vi "read_idcode.vi"() -> ()   [LabVIEW 2017]
panel:
  out "字符串":string
  out "数值":i32=2
  out "Out":u8=67 format="%.0x"
  out "received string 2":string="C"
  out "received string":string
  in  "数组":string[](array[string])=[":\u0005\u0000\u0000\u0000\u001f\u0000", ":\u0004\u0000\u0000\u0000\u0002\u0000", ": \u0000\u0000\u0000\u0000\u0000"]
  out "错误输出":errorcluster
  in  "address":string="192.168.10.20"
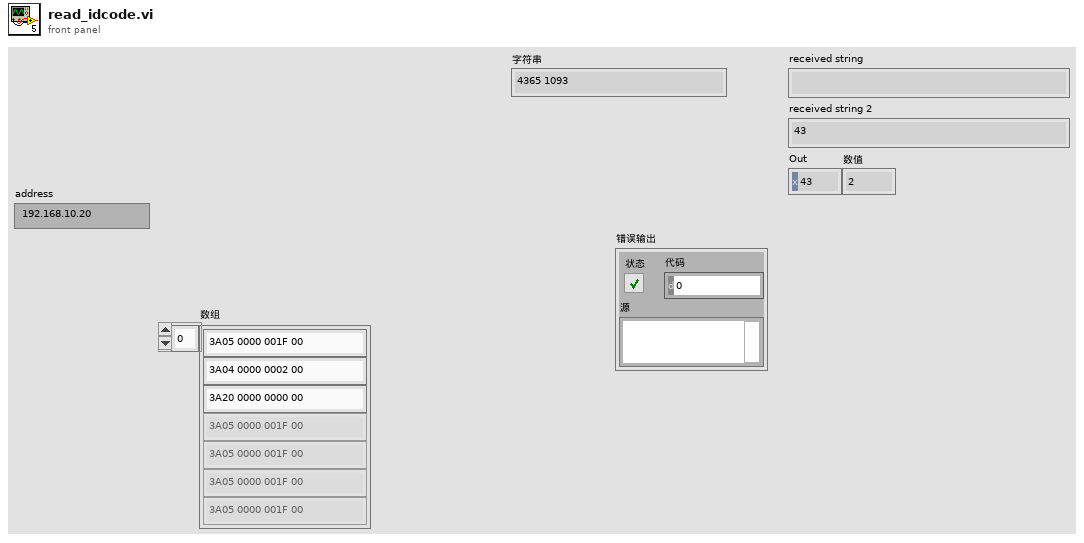
[diagram p1: front panel]
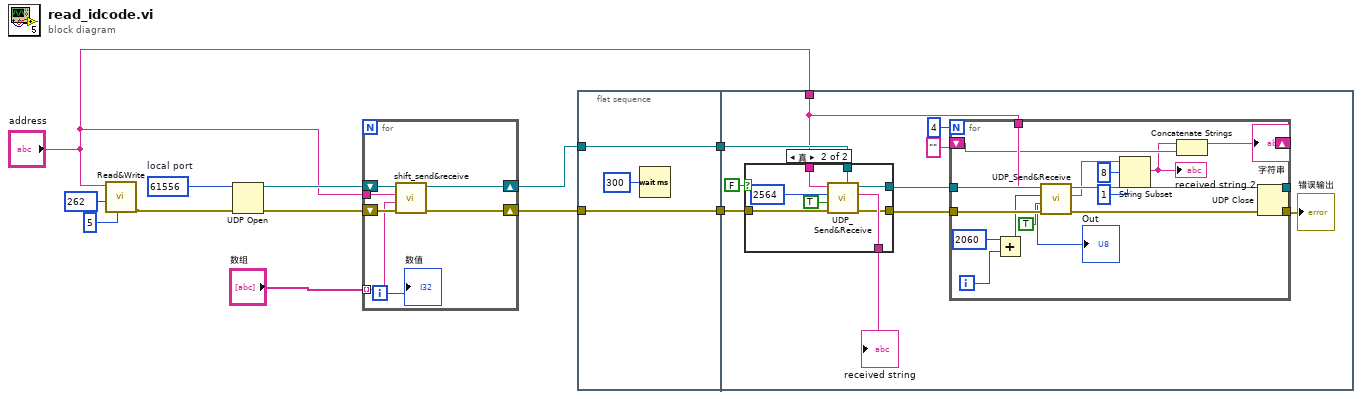
[diagram p0: block diagram]
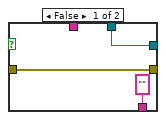
[diagram p2: hidden frame]
diagram:
  w12 = u16 61556  # local port
  n1 = call "Read&Write.vi"("In"=u8 5, "Address"=u32 262, "address"="address") -> ("error out"=w9:errorcluster)  [unwired: 7 in, 1 out]
  n2 = UDP Open(8:w9, 11:w12) -> (port=w8:refnum<k16>, 0:w7:errorcluster)  [unwired: 3 in, 1 out]
  n3 = for {
    tunnel: "address" -> [w17]
    shift-right: [w15] -> w5
    shift-left: w8 -> [w19]
    shift-right: [w16] -> w4
    shift-left: w7 -> [w18]
    tunnel: "数组" -> [w14] mode=indexing
    i -> [w13]
    n4 = call "shift_send&receive.vi"("error in"=w18, "shift string"=w14, "ip address"=w17, "port"=w19) -> ("error out"=w16:errorcluster, "connection ID 2"=w15:refnum<k16>)  [unwired: 6 in]
    "数值" <- w13
  }
  n5 = flat-sequence {
    tunnel: w4 -> [w21]
    tunnel: w5 -> [w22]
    tunnel: [w22] -> w2
    tunnel: [w21] -> w1
    tunnel: "address" -> [w23]
    tunnel: w2 -> [w35]
    tunnel: w1 -> [w34]
    frame #0 {
      n6 = Wait (ms)(milliseconds to wait=u32 300 ("等待时间（毫秒）")) -> ()  [unwired: 1 out]
    }
    frame #1 {
      n7 = case shown="真" FALSE {
        tunnel: w35 -> [w54 w62]
        tunnel: w34 -> [w53 w61]
        tunnel: ["" ("received string") w58] -> w33
        tunnel: [w54 w57] -> w32
        tunnel: [w53 w56] -> w31
        tunnel: w23 -> [_ w55]
        frame False {
        }
        frame True {
          n8 = call "UDP_Send&Receive.vi"("connection ID"=w62, "error in (no error)"=w61, "Read (TRUE)"=TRUE, "Address"=u32 2564, "IP address"=w55) -> ("error out"=w56:errorcluster, "received string"=w58:string, "connection ID out"=w57:refnum<k16>)  [unwired: 2 in, 1 out]
        }
      }
      "received string" <- w33
      n9 = for {
        N: 4 -> [_]
        tunnel: w32 -> [w51]
        tunnel: w31 -> [w50]
        tunnel: w23 -> [w49]
        shift-right: [w43] -> w27
        shift-left: "" -> [w42]
        tunnel: [w41] -> w25
        tunnel: [w40] -> w24
        i -> [w44]
        n10 = Add(x=u32 2060 ("Address"), y=w44) -> (x+y=w45:u32)
        n11 = call "UDP_Send&Receive.vi"("connection ID"=w51, "error in (no error)"=w50, "Read (TRUE)"=TRUE, "Address"=w45, "IP address"=w49) -> ("error out"=w41:errorcluster, "Out"=→"Out":u8, "received string"=w39:string, "connection ID out"=w40:refnum<k16>)  [unwired: 2 in]
        n12 = String Subset(string=w39, offset (0)=8 ("偏移量(0)"), length (rest)=1 ("长度（剩余）")) -> (substring=w38:string)
        "received string 2" <- w38
        n13 = Concatenate Strings(w38, w42) -> (w43:string)
      }
      "字符串" <- w27
      n14 = UDP Close(connection ID=w24, 8:w25) -> (error out=→"错误输出":errorcluster)  [unwired: 1 out]
    }
  }
